vi "GetStreamStatus.vi"(0 "reference in":refnum<class "SuperNS.lvclass">, 5 "error in":errorcluster) -> (14 "reference out":refnum<class "SuperNS.lvclass">, 16 "StreamStatus":T1, 17 "R/W Error":bool, 18 "NS Created":bool, 19 "error out":errorcluster)   [LabVIEW 2020, in "SuperNS.lvclass"]
doc: "Copyright © 2008 - 2024 VI Technologies B.V. \nALL RIGHTS RESERVED\n\nReturn the current status of the network stream endpoint (if a stream is active) in <b>StreamStatus</b> and the SuperNS internal status bits <b>R/W Error</b> and <b>NS Created</b>.\n\nIf <b>R/W Error</b> is true, the SuperNS will attempt to reconnect in the background.\nIf <b>NS Created</b> is true, the network stream should be ready to use."
uses:
  SuperNS.lvclass
  StreamStatus.ctl
  SuperNS.lvclass/SuperNS.ctl
  <resource>/objmgr/ni.dex.rc
panel:
  # "Copyright (c) 2024, VI Technologies B.V.\nAll rights reserved.\n\nRedistribution and use in source and binary forms, with or without modification, are permitted provided that \nthe following conditions are met:\n\n * Redistributions of source code must retain the above copyright notice, this list of conditions and the \nfollowing disclaimer.\n * Redistributions in binary form must reproduce the above copyright notice, this list of conditions and the \nfollowing disclaimer in the documentation and/or other materials provided with the distribution.\n * Neither the name of VI Technologies B.V. nor the names of its contributors may be used to endorse or \npromote products derived from this software without specific prior written permission.\n\nTHIS SOFTWARE IS PROVIDED BY THE COPYRIGHT HOLDERS AND CONTRIBUTORS \"AS IS\" AND ANY EXPRESS OR \nIMPLIED WARRANTIES, INCLUDING, BUT NOT LIMITED TO, THE IMPLIED WARRANTIES OF MERCHANTABILITY \nAND FITNESS FOR A PARTICULAR PURPOSE ARE DISCLAIMED. IN NO EVENT SHALL THE COPYRIGHT OWNER OR \nCONTRIBUTORS BE LIABLE FOR ANY DIRECT, INDIRECT, INCIDENTAL, SPECIAL, EXEMPLARY, OR CONSEQUENTIAL \nDAMAGES (INCLUDING, BUT NOT LIMITED TO, PROCUREMENT OF SUBSTITUTE GOODS OR SERVICES; LOSS OF \nUSE, DATA, OR PROFITS; OR BUSINESS INTERRUPTION) HOWEVER CAUSED AND ON ANY THEORY OF LIABILITY, \nWHETHER IN CONTRACT, STRICT LIABILITY, OR TORT (INCLUDING NEGLIGENCE OR OTHERWISE) ARISING IN ANY \nWAY OUT OF THE USE OF THIS SOFTWARE, EVEN IF ADVISED OF THE POSSIBILITY OF SUCH DAMAGE.\n\nFor more information, please visit https://www.vi-tech.nl or contact us at info@vi-tech.nl"
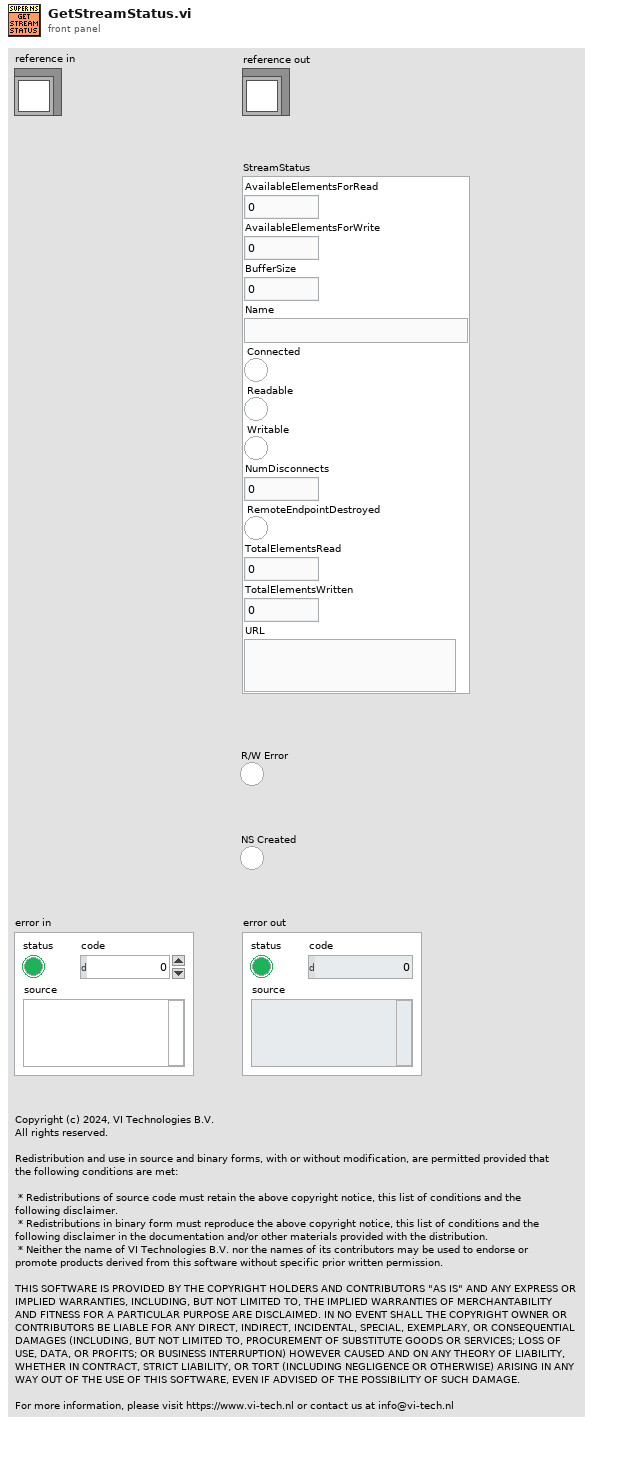
[diagram p1: front panel]
types:
  T1 = typedef "SuperNS.lvclass/StreamStatus.ctl" = cluster{"AvailableElementsForRead":i32, "AvailableElementsForWrite":i32, "BufferSize":i32, "Name":string, "Connected":bool, "Readable":bool, "Writable":bool, "NumDisconnects":u32, "RemoteEndpointDestroyed":bool, "TotalElementsRead":u64, "TotalElementsWritten":u64, "URL":string}
  T2 = typedef "SuperNS.lvclass/ObjectAttributes.ctl" = cluster{"NSName":string, "RemoteEP_URL":string, "BufferSize":i32, "Element Allocation Mode":T3, "ConnLost Timeout":i32, "Writer":bool, "ReadDataEvent":string, "FlushAfterWrite":bool, "Thread":cluster{"VI Refnum":refnum<vi>, "Started Notifier":refnum<notifier>, "Stopped Notifier":refnum<notifier>, "CmdEvent":refnum<user-event>}, "Endpoint":refnum<k21>, "R/W Error":bool, "Flush Wait Condition":T4, "DataReadEvent":refnum<user-event>, "NS Created":bool, "BG ConnCheck/Read period":i32, "ErrorEvent":refnum<user-event>}
  T3 = typedef "Stream Element Allocation Mode.ctl" = u32
  T4 = typedef "Flush And Wait Empty Condition.ctl" = u8
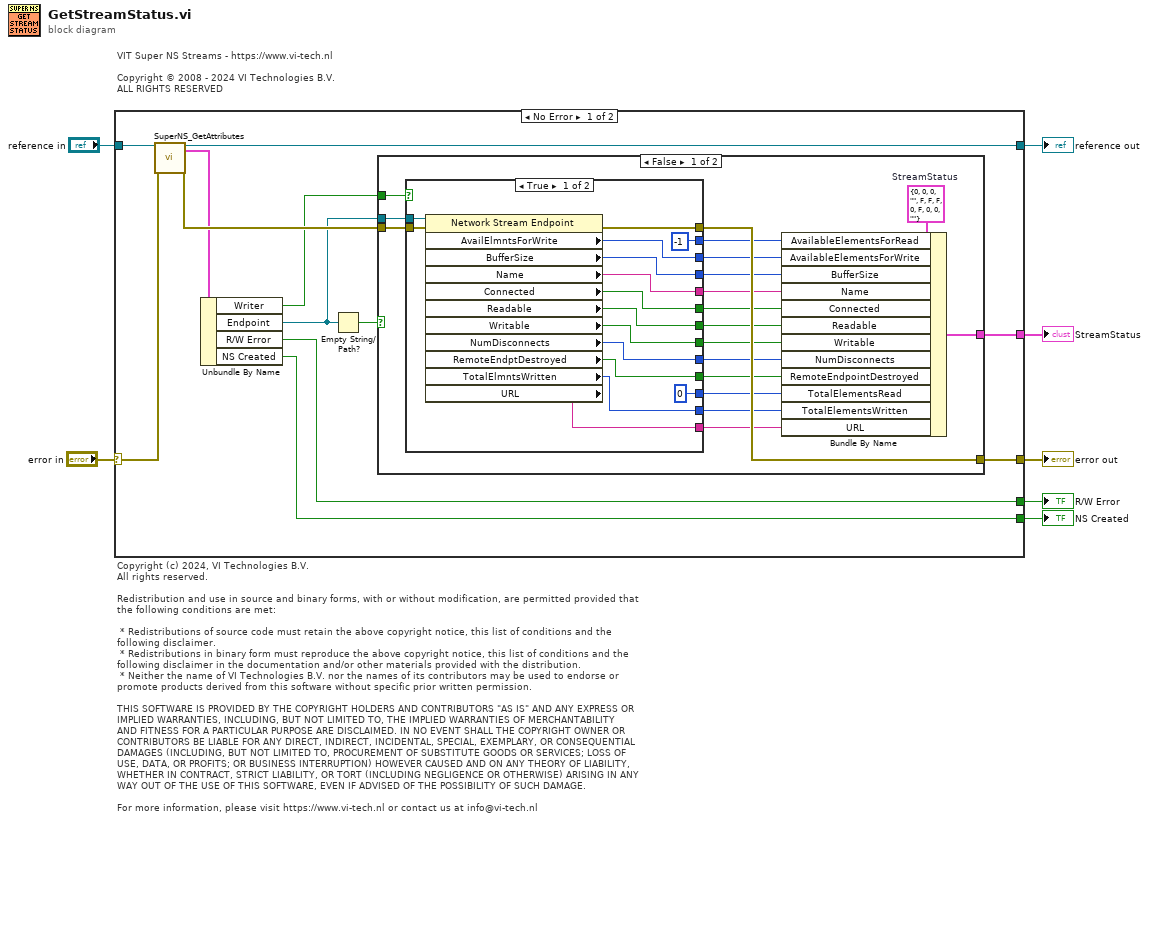
[diagram p0: block diagram]
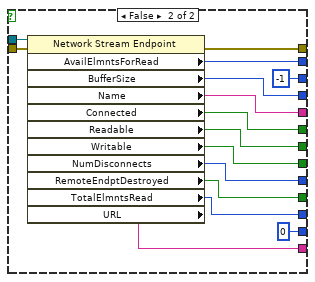
[diagram p2: hidden frame]
diagram:
  # "VIT Super NS Streams - https://www.vi-tech.nl\n\nCopyright © 2008 - 2024 VI Technologies B.V. \nALL RIGHTS RESERVED"
  # "Copyright (c) 2024, VI Technologies B.V.\nAll rights reserved.\n\nRedistribution and use in source and binary forms, with or without modification, are permitted provided that \nthe following conditions are met:\n\n * Redistributions of source code must retain the above copyright notice, this list of conditions and the \nfollowing disclaimer.\n * Redistributions in binary form must reproduce the above copyright notice, this list of conditions and the \nfollowing disclaimer in the documentation and/or other materials provided with the distribution.\n * Neither the name of VI Technologies B.V. nor the names of its contributors may be used to endorse or \npromote products derived from this software without specific prior written permission.\n\nTHIS SOFTWARE IS PROVIDED BY THE COPYRIGHT HOLDERS AND CONTRIBUTORS \"AS IS\" AND ANY EXPRESS OR \nIMPLIED WARRANTIES, INCLUDING, BUT NOT LIMITED TO, THE IMPLIED WARRANTIES OF MERCHANTABILITY \nAND FITNESS FOR A PARTICULAR PURPOSE ARE DISCLAIMED. IN NO EVENT SHALL THE COPYRIGHT OWNER OR \nCONTRIBUTORS BE LIABLE FOR ANY DIRECT, INDIRECT, INCIDENTAL, SPECIAL, EXEMPLARY, OR CONSEQUENTIAL \nDAMAGES (INCLUDING, BUT NOT LIMITED TO, PROCUREMENT OF SUBSTITUTE GOODS OR SERVICES; LOSS OF \nUSE, DATA, OR PROFITS; OR BUSINESS INTERRUPTION) HOWEVER CAUSED AND ON ANY THEORY OF LIABILITY, \nWHETHER IN CONTRACT, STRICT LIABILITY, OR TORT (INCLUDING NEGLIGENCE OR OTHERWISE) ARISING IN ANY \nWAY OUT OF THE USE OF THIS SOFTWARE, EVEN IF ADVISED OF THE POSSIBILITY OF SUCH DAMAGE.\n\nFor more information, please visit https://www.vi-tech.nl or contact us at info@vi-tech.nl"
  n1 = case shown="No Error" "error in" {
    selector: "error in" -> [w19 w70]
    tunnel: [w17 w70] -> w2
    tunnel: [w15 w69] -> w6
    tunnel: "reference in" -> [w16 w69]
    tunnel: [w14 _] -> w5
    tunnel: [w9 _] -> w4
    tunnel: [w8 _] -> w3
    frame No Error {
      n2 = call "SuperNS_GetAttributes.vi"("reference in"=w16, "error in"=w19) -> ("reference out"=w15:refnum<class "SuperNS.lvclass">, "Data"=w12:T2, "error out"=w18:errorcluster)  [unwired: 14 in, 1 out]
      n3 = Unbundle By Name(w12) -> ("Writer"=w11:bool, "Endpoint"=w10:refnum<k21>, "R/W Error"=w9:bool, "NS Created"=w8:bool)
      n4 = Empty String/Path?(string/path=w10) -> (empty?=w13:bool)
      n5 = case shown="False" w13 {
        tunnel: w18 -> [w37 w68]
        tunnel: [w36 w68] -> w17
        tunnel: [w22 _] -> w14
        tunnel: w11 -> [w21 _]
        tunnel: w10 -> [w20 _]
        frame False {
          w23 = T1 {"AvailableElementsForRead"=0, "AvailableElementsForWrite"=0, "BufferSize"=0, "Name"="", "Connected"=FALSE, "Readable"=FALSE, "Writable"=FALSE, "NumDisconnects"=0, "RemoteEndpointDestroyed"=FALSE, "TotalElementsRead"=0, "TotalElementsWritten"=0, "URL"=""}  # StreamStatus
          n6 = case shown="True" w21 {
            tunnel: w20 -> [w50 w65]
            tunnel: w37 -> [w52 w67]
            tunnel: [w51 w66] -> w36
            tunnel: [-1 ("AvailElmntsForRead") w64] -> w35
            tunnel: [w49 -1 ("AvailElmntsForWrite")] -> w34
            tunnel: [w48 w63] -> w33
            tunnel: [w47 w62] -> w32
            tunnel: [w46 w61] -> w31
            tunnel: [w45 w60] -> w30
            tunnel: [w44 w59] -> w29
            tunnel: [w43 w58] -> w28
            tunnel: [w42 w57] -> w27
            tunnel: [u64 0 ("TotalElmntsRead") w56] -> w26
            tunnel: [w41 u64 0 ("TotalElmntsWritten")] -> w25
            tunnel: [w40 w55] -> w24
            frame True {
              n7 = property class="Network Stream Endpoint"(reference=w50, error in=w52) -> (error out=w51:errorcluster, "AvailElmntsForWrite"=w49:i32, "BufferSize"=w48:i32, "Name"=w47:string, "Connected"=w46:bool, "Readable"=w45:bool, "Writable"=w44:bool, "NumDisconnects"=w43:u32, "RemoteEndptDestroyed"=w42:bool, "TotalElmntsWritten"=w41:u64, "URL"=w40:string)  [unwired: 1 out]
            }
            frame False {
              n8 = property class="Network Stream Endpoint"(reference=w65, error in=w67) -> (error out=w66:errorcluster, "AvailElmntsForRead"=w64:i32, "BufferSize"=w63:i32, "Name"=w62:string, "Connected"=w61:bool, "Readable"=w60:bool, "Writable"=w59:bool, "NumDisconnects"=w58:u32, "RemoteEndptDestroyed"=w57:bool, "TotalElmntsRead"=w56:u64, "URL"=w55:string)  [unwired: 1 out]
            }
          }
          n9 = Bundle By Name(cluster=w23, "AvailableElementsForRead"=w35, "AvailableElementsForWrite"=w34, "BufferSize"=w33, "Name"=w32, "Connected"=w31, "Readable"=w30, "Writable"=w29, "NumDisconnects"=w28, "RemoteEndpointDestroyed"=w27, "TotalElementsRead"=w26, "TotalElementsWritten"=w25, "URL"=w24) -> (w22:T1)
        }
        frame True {
        }
      }
    }
    frame Error {
    }
  }
  "reference out" <- w6
  "StreamStatus" <- w5
  "R/W Error" <- w4
  "NS Created" <- w3
  "error out" <- w2
